vi "Initialisation_Tester_Parameter.vi"() -> (1 "Pressure(Pa)":dbl, 3 "Initialisation_Tester_Parameter":dbl[](array[numeric]))   [LabVIEW 2017]
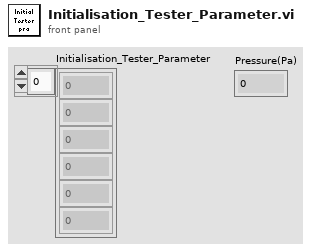
[diagram p1: front panel]
types:
  T1 = typedef "HD Config.ctl" = cluster{" PC":cluster{"PC Address":u8[], "PC Port":i32}, "FCO":cluster{"COM":refnum<visa-resource-name>, "Baudrate":u32}, "DC Power ":cluster{"COM":refnum<visa-resource-name>, "Baudrate":u32}, "PW3336":cluster{"COM":refnum<visa-resource-name>, "Baudrate":u32}, "Lefoo":cluster{"COM":refnum<visa-resource-name>, "Baudrate":u32}, "AI Model":cluster{"COM":refnum<visa-resource-name>, "Baudrate":u32}, "DIPC":cluster{"COM":refnum<visa-resource-name>}, "RFID":cluster{"IP Address":string, "Port":u16, "Retry":u16}, "Motor":cluster{"COM":refnum<visa-resource-name>, "Baudrate":u32}, "Fail_resume_mode":bool, "GRR":bool}
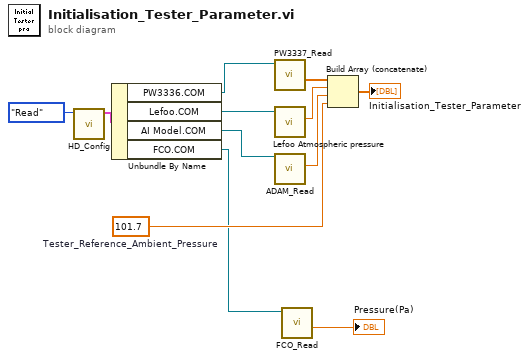
[diagram p0: block diagram]
diagram:
  w5 = 101.7  # Tester_Reference_Ambient_Pressure
  n1 = call "HD_Config.vi"("Step"=enum16{"Initial", "Write", "Read"}."Read") -> ("HD Config out"=w11:T1)  [unwired: 9 in, 1 out]
  n2 = Unbundle By Name(w11) -> ("PW3336.COM"=w10:refnum<visa-resource-name>, "Lefoo.COM"=w9:refnum<visa-resource-name>, "AI Model.COM"=w8:refnum<visa-resource-name>, "FCO.COM"=w2:refnum<visa-resource-name>)
  n3 = call "PW3337_Read.vi"("VISA resource name"=w10) -> ("Measurement out"=w7:dbl[])  [unwired: 7 in, 3 out]
  n4 = call "Lefoo Atmospheric pressure.vi"("VISA resource name"=w9) -> ("Atmospheric pressure"=w6:dbl)  [unwired: 8 in, 2 out]
  n5 = call "ADAM_Read.vi"("VISA resource name"=w8) -> ("temperature"=w3:dbl)  [unwired: 7 in, 3 out]
  n6 = call "FCO_Read.vi"("VISA in"=w2) -> ("Pressure(Pa)"=→"Pressure(Pa)":dbl)  [unwired: 7 in, 3 out]
  n7 = Build Array (concatenate)(w7, w6, w3, w5) -> (→"Initialisation_Tester_Parameter":dbl[])
